vi "Picolog Setup Channels.vi"(8 "Error In":errorcluster, 9 "Configurations":T1[](array[typedef]) items=["B"=98, "E"=101, "J"=106, "K"=107, "N"=110, "R"=114, "S"=115, "T"=116, "Voltage"=120, "Internal"=0, "Off"=32], 11 "Instrument Handle":i16) -> (0 "Error Out":errorcluster, 2 "Channels":i16[](array[numeric]), 3 "Instrument Handle Out":i16)   [LabVIEW 2017]
uses:
  Controls/Thermocouple.ctl
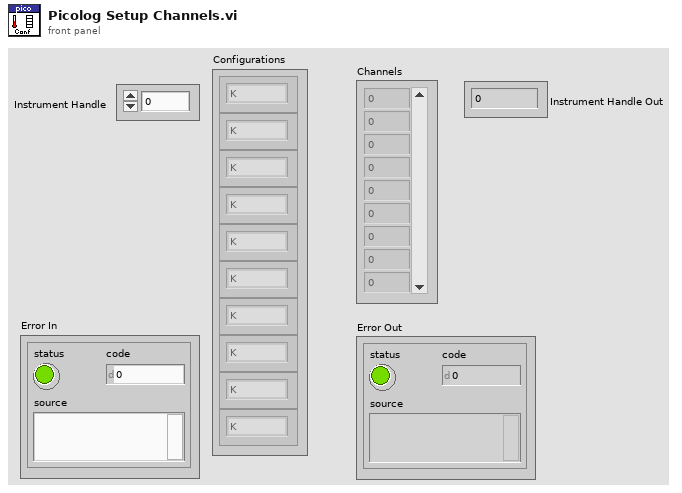
[diagram p1: front panel]
types:
  T1 = typedef "Thermocouple.ctl" = i8
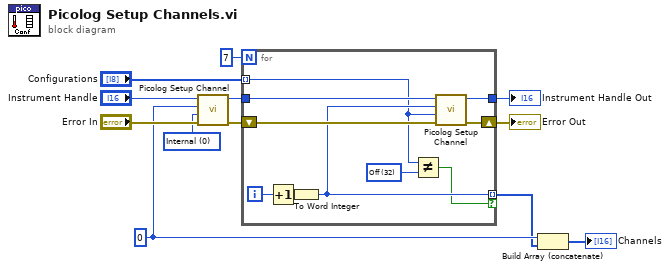
[diagram p0: block diagram]
diagram:
  w4 = T1 0 items=["B"=98, "E"=101, "J"=106, "K"=107, "N"=110, "R"=114, "S"=115, "T"=116, "Voltage"=120, "Internal"=0, "Off"=32] ("Configuration")
  w3 = i16 0 ("Channel")
  n1 = call "Picolog Setup Channel.vi"("Error In"="Error In", "Termocouple Type"=w4, "Channel"=w3, "Instrument Handle In"="Instrument Handle") -> ("Error Out"=w6:errorcluster, "Instrument Handle Out"=w8:i16)  [unwired: 6 in]
  n2 = for {
    N: 7 -> [_]
    tunnel: w8 -> [w22]
    shift-right: [w21] -> w11
    shift-left: w6 -> [w20]
    tunnel: [w19] -> w10
    tunnel: "Configurations" -> [w15] mode=indexing
    tunnel: [w16] -> w2 mode=indexing if=w14
    i -> [w18]
    w13 = T1 32 items=["B"=98, "E"=101, "J"=106, "K"=107, "N"=110, "R"=114, "S"=115, "T"=116, "Voltage"=120, "Internal"=0, "Off"=32] ("y")
    n3 = Increment(x=w18) -> (x+1=w17:i32)
    n4 = To Word Integer(number=w17) -> (16bit integer=w16:i16)
    n5 = Not Equal?(x=w15, y=w13) -> (x != y?=w14:bool)
    n6 = call "Picolog Setup Channel.vi"("Error In"=w20, "Termocouple Type"=w15, "Channel"=w16, "Instrument Handle In"=w22) -> ("Error Out"=w21:errorcluster, "Instrument Handle Out"=w19:i16)  [unwired: 6 in]
  }
  "Error Out" <- w11
  "Instrument Handle Out" <- w10
  n7 = Build Array (concatenate)(w3, w2) -> (→"Channels":i16[])
